vi "Get Sensitivity.vi"(7 "dDev":dbl, 8 "error in (no error)":errorcluster, 9 "nRefSens":i32, 10 "nSens":i32, 11 "nSensorIP":u32) -> (0 "error out":errorcluster, 1 "nRefSens out":i32, 2 "nSens out":i32, 3 "function return":i32, 5 "dDev out":dbl)   [LabVIEW 2017, in "imgAcquisition.lvlib"]
doc: "DLLFunction int __stdcall ImageCapGetSensitivity(unsigned int nSensorIP, int* nSens, int* nRefSens, double* dDev);"
uses:
  imgAcquisition.lvlib
  lib/ImageCaptureDLL.dll
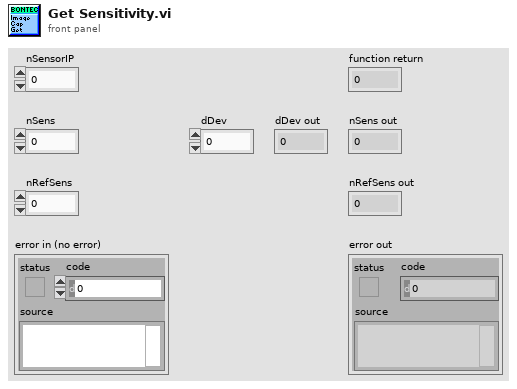
[diagram p1: front panel]
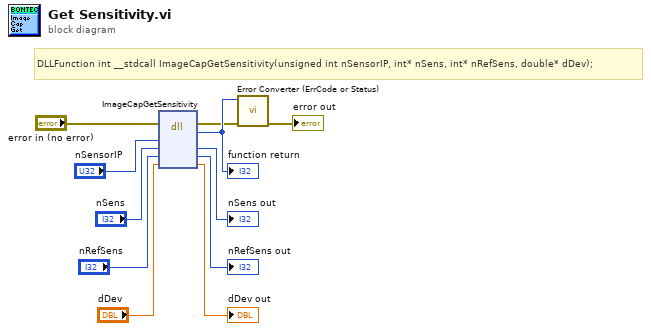
[diagram p0: block diagram]
diagram:
  # "DLLFunction int __stdcall ImageCapGetSensitivity(unsigned int nSensorIP, int* nSens, int* nRefSens, double* dDev);"
  n1 = dll-call lib="F:/BonTechFlatPanelLVDriver/lib/ImageCaptureDLL.*" fn="ImageCapGetSensitivity"(error in="error in (no error)", "nSensorIP"="nSensorIP", "nSens"="nSens", "nRefSens"="nRefSens", "dDev"="dDev") -> (error out=w2:errorcluster, w11:i32, "nSens"=→"nSens out":i32, "nRefSens"=→"nRefSens out":i32, "dDev"=→"dDev out":dbl)  [unwired: 3 in, 1 out]
  "function return" <- w11
  n2 = call "Error Converter (ErrCode or Status).vi"("error in (no error)"=w2, "error code"=w11) -> ("error out"=→"error out":errorcluster)  [unwired: 9 in]
